vi "Asyncronous TDCReader launcher.vi"(8 "error in":errorcluster, 9 "hitRateWarning ChannelHits":refnum<vi>, 10 "FastRead cluster":T2, 11 "Read Cluster":T3) -> (0 "error out":errorcluster, 1 "Sorter Refnum":refnum<vi>, 2 "TDCFastRead Refnum":refnum<vi>, 3 "TDCRead Refnum":refnum<vi>)   [LabVIEW 2016]
uses:
  HPTDC Driver Library Folder/Library files/Typedefs/TDCManagerRefnum.ctl
  HPTDC Driver Library Folder/Library files/Typedefs/TDCManager.ctl
  C:/Users/CRT Controller/CRTC Labview Application/Source/HPTDC Driver Library Folder/Library files/hptdc_net4_3.7.0_x64.dll
  HPTDC Driver Library Folder/Library files/hptdc_net4_3.7.0_x64.dll
  HPTDC Driver Library Folder/HPTDC Driver Library.lvlib
panel:
  # "This VI launches asynchronously the fast TDC reader and the normal TDC reader, as well as the \nTDCHit sorter VI."
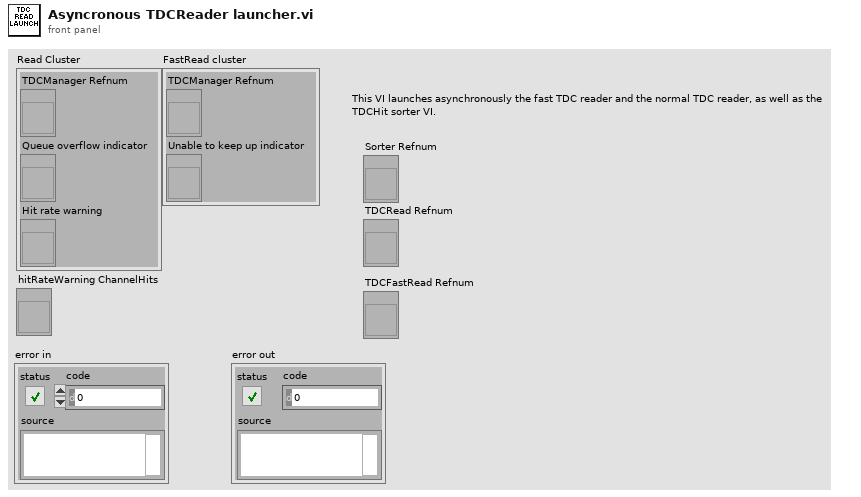
[diagram p1: front panel]
types:
  T1 = typedef "TDCManagerRefnum.ctl" = refnum<vi>
  T2 = cluster{"TDCManager Refnum":T1, "Unable to keep up indicator":refnum<vi>}
  T3 = cluster{"TDCManager Refnum":T1, "Queue overflow indicator":refnum<vi>, "Hit rate warning":refnum<vi>}
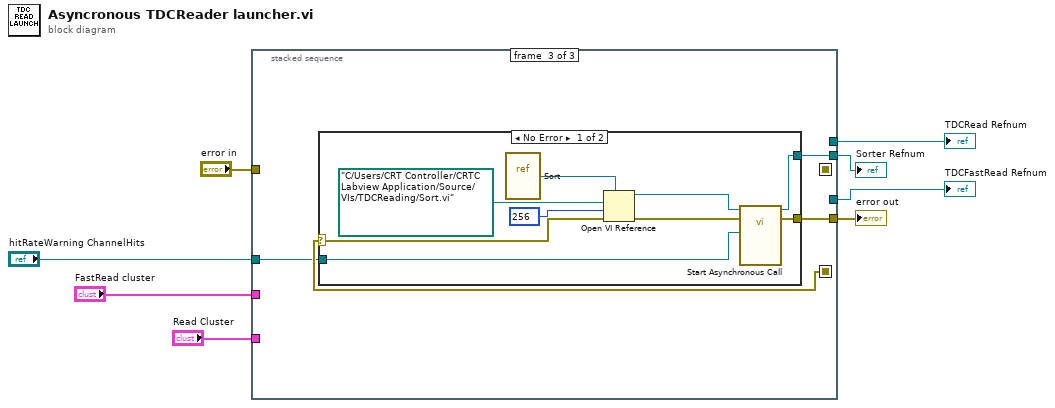
[diagram p0: block diagram]
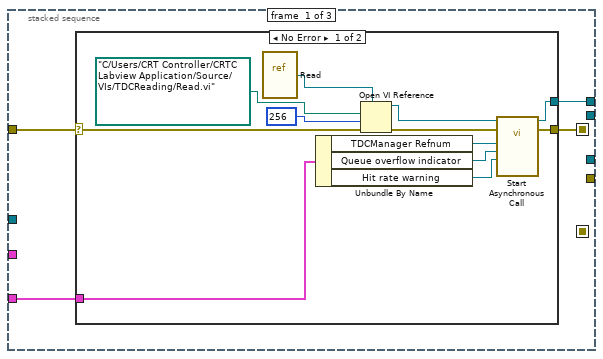
[diagram p2: hidden frame]
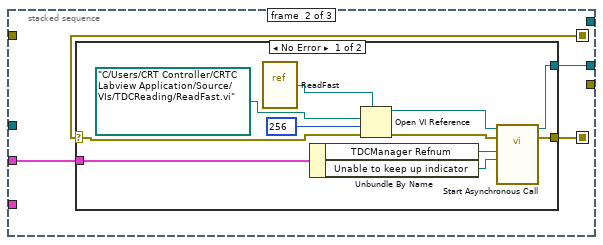
[diagram p4: hidden frame]
diagram:
  n1 = stacked-sequence {
    seq-local: [w11 _ _] -> [_ w29 _]
    seq-local: [_ w27 _] -> [_ _ w45]
    tunnel: "Read Cluster" -> [w12 _ _]
    tunnel: "error in" -> [w10 _ _]
    tunnel: "FastRead cluster" -> [_ w28 _]
    tunnel: [_ _ w44] -> w7
    tunnel: "hitRateWarning ChannelHits" -> [_ _ w43]
    tunnel: [_ _ w42] -> w3
    tunnel: [w9 _ _] -> w2
    tunnel: [_ w26 _] -> w1
    frame #0 {
      n2 = case shown="No Error" w10 {
        selector: w10 -> [w19 w25]
        tunnel: w12 -> [w20 _]
        tunnel: [w16 w25] -> w11
        tunnel: [w15 _] -> w9
        frame No Error {
          n3 = vi-ref "Read.vi"() -> (w22:refnum<vi>)
          n4 = Unbundle By Name(w20) -> ("TDCManager Refnum"=w13:T1, "Queue overflow indicator"=w18:refnum<vi>, "Hit rate warning"=w17:refnum<vi>)
          n5 = Open VI Reference(type specifier VI Refnum (for type only)=w22, vi path=path "C:/Users/CRT Controller/CRTC Labview Application/Source/VIs/TDCReading/Read.vi", options=256, error in (no error)=w19) -> (vi reference=w14:refnum<vi>, error out=w21:errorcluster)  [unwired: 2 in]
          n6 = call-by-ref "Start Asynchronous Call"(reference=w14, error in=w21, "Hit rate warning"=w17, "Queue overflow indicator"=w18, "TDCManager refnum"=w13) -> (reference out=w15:refnum<vi>, error out=w16:errorcluster)  [unwired: 8 in, 1 out]
        }
        frame Error {
        }
      }
    }
    frame #1 {
      n7 = case shown="No Error" w29 {
        selector: w29 -> [w34 w41]
        tunnel: w28 -> [w35 _]
        tunnel: [w32 w41] -> w27
        tunnel: [w31 _] -> w26
        frame No Error {
          n8 = vi-ref "ReadFast.vi"() -> (w38:refnum<vi>)
          n9 = Unbundle By Name(w35) -> ("TDCManager Refnum"=w30:T1, "Unable to keep up indicator"=w33:refnum<vi>)
          n10 = Open VI Reference(type specifier VI Refnum (for type only)=w38, vi path=path "C:/Users/CRT Controller/CRTC Labview Application/Source/VIs/TDCReading/ReadFast.vi", options=256, error in (no error)=w34) -> (vi reference=w37:refnum<vi>, error out=w36:errorcluster)  [unwired: 2 in]
          n11 = call-by-ref "Start Asynchronous Call"(reference=w37, error in=w36, "Unable to keep up indicator"=w33, "TDCManager"=w30) -> (reference out=w31:refnum<vi>, error out=w32:errorcluster)  [unwired: 9 in, 1 out]
        }
        frame Error {
        }
      }
    }
    frame #2 {
      n12 = case shown="No Error" w45 {
        selector: w45 -> [w49 w55]
        tunnel: [w47 w55] -> w44
        tunnel: w43 -> [w48 _]
        tunnel: [w46 _] -> w42
        frame No Error {
          n13 = vi-ref "Sort.vi"() -> (w52:refnum<vi>)
          n14 = Open VI Reference(type specifier VI Refnum (for type only)=w52, vi path=path "C:/Users/CRT Controller/CRTC Labview Application/Source/VIs/TDCReading/Sort.vi", options=256, error in (no error)=w49) -> (vi reference=w51:refnum<vi>, error out=w50:errorcluster)  [unwired: 2 in]
          n15 = call-by-ref "Start Asynchronous Call"(reference=w51, error in=w50, "hitRateWarning ChannelHits"=w48) -> (reference out=w46:refnum<vi>, error out=w47:errorcluster)  [unwired: 10 in, 1 out]
        }
        frame Error {
        }
      }
    }
  }
  "error out" <- w7
  "Sorter Refnum" <- w3
  "TDCRead Refnum" <- w2
  "TDCFastRead Refnum" <- w1
